vi "Get_Sampling_Info.vi"() -> (0 "Channel Values":string[](array[string]), 1 "Channel Names":string[](array[string]))   [LabVIEW 2011]
uses:
  Anemometry Sub Vis/Controls/Instrument_Array.ctl
  Anemometry Sub Vis/Globals/Meas_global.vi
  Anemometry Sub Vis/Globals/LDA_meas_global_1.vi
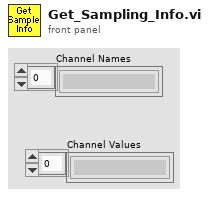
[diagram p1: front panel]
types:
  T1 = typedef "Instrument_Array.ctl" = enum16{"PWA", "LDA", "Analogue"}
  T2 = typedef "Analysis_info_cluster.ctl" = cluster{"Colour":u32, "Inst type":T3, "Inst name":string, "Symbol":string, "Code name":string, "Extra Info":string, "Inst Array":T1, "Extra Titles":string[], "Extra Values":string[], "Eng Values":dbl[], "Time (ms)":dbl[], "Voltage":dbl[], "U":dbl, "u^2":dbl, "u^3":dbl, "u^4":dbl, "Skew_u":dbl, "Kurt_u":dbl, "Sd Error in Mean":dbl, "% u'/U":dbl, "X":dbl, "Y":dbl, "Z":dbl, "Spectra":T4, "Autocorrelation":T4, "Timescale integral to 25%":dbl, "Sd Error in Variance":dbl, "Calib File":path, "Calib Constants":dbl[], "Histogram":T4, "Output Position":bool, "Full Stats":bool, "Weighting":dbl[], "Av Sampling Rate":dbl, "Av No of Samples":dbl, "Total Meas Time (s)":dbl}
  T3 = typedef "Inst_type.ctl" = enum16{"Propeller anemometer", "Raw voltage", "Pressure Transducer", "Pitot-static tube", "Preston tube", "Hot wire", "Cross wire 1", "Cross wire 2", "Generic Linear", "Generic Polynomial", "Generic BackPoly", "Fast FID", "Thermocouple", "Cold wire", "Pulsed Wire", "LDA Vel", "LDA Tran time", "LDA Arr time"}
  T4 = typedef "XY_Plot_Cluster.ctl" = cluster{"First Name":string, "Second Name":string, "X axis name":string, "Y axis name":string, "X array":dbl[], "Y array":dbl[]}
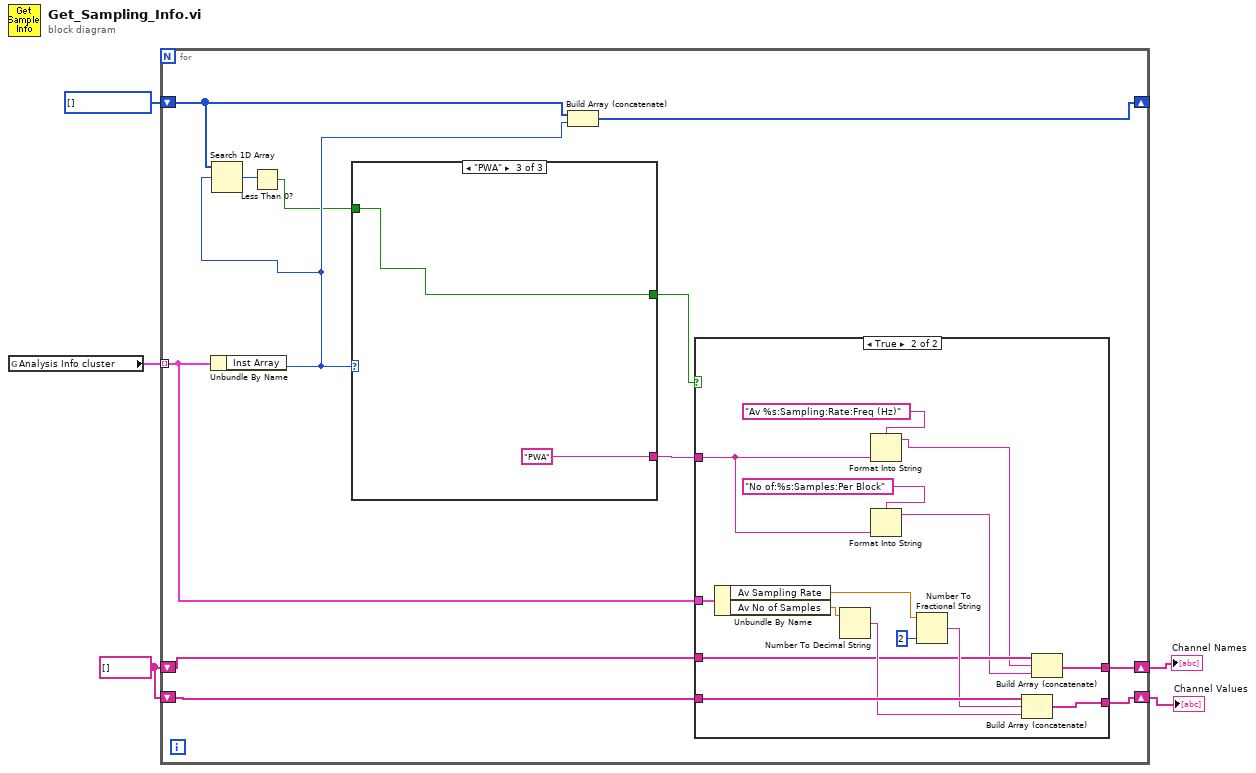
[diagram p0: block diagram]
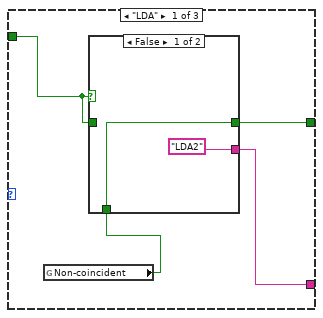
[diagram p3: hidden frame]
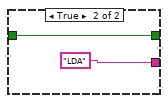
[diagram p4: hidden frame]
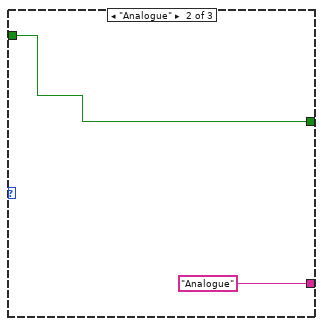
[diagram p5: hidden frame]
diagram:
  w3 = string[] []
  w4 = T1[] [] items=["PWA", "LDA", "Analogue"]
  n1 = global read "Meas_global.vi" "Analysis Info cluster"() -> (w5:T2[])
  n2 = for {
    shift-right: [w17] -> _
    shift-left: w4 -> [w16]
    tunnel: w5 -> [w11] mode=indexing
    shift-right: [w6] -> w1
    shift-left: w3 -> [w7]
    shift-right: [w8] -> w2
    shift-left: w3 -> [w9]
    n3 = Unbundle By Name(w11) -> ("Inst Array"=w15:T1)
    n4 = Search 1D Array(1D array=w16, element=w15) -> (index of element=w14:i32)  [unwired: 1 in]
    n5 = Less Than 0?(x=w14) -> (x < 0?=w13:bool)
    n6 = case shown="\"PWA\"" w15 {
      tunnel: w13 -> [w37 w44 w46]
      tunnel: [w38 w44 w46] -> w12
      tunnel: [w36 "Analogue" "PWA"] -> w10
      frame "LDA" {
        n7 = global read "LDA_meas_global_1.vi" "Non-coincident"() -> (w35:bool)
        n8 = case shown="False" w37 {
          tunnel: [w40 w42] -> w38
          tunnel: w37 -> [_ w42]
          tunnel: ["LDA2" "LDA"] -> w36
          tunnel: w35 -> [w40 _]
          frame False {
          }
          frame True {
          }
        }
      }
      frame "Analogue" {
      }
      frame "PWA" {
      }
    }
    n9 = Build Array (concatenate)(w16, w15) -> (w17:T1[])
    n10 = case shown="True" w12 {
      tunnel: w11 -> [_ w34]
      tunnel: w10 -> [_ w21]
      tunnel: w9 -> [w18 w31]
      tunnel: [w18 w30] -> w8
      tunnel: w7 -> [w19 w25]
      tunnel: [w19 w24] -> w6
      frame False {
      }
      frame True {
        n11 = Unbundle By Name(w34) -> ("Av Sampling Rate"=w28:dbl, "Av No of Samples"=w27:dbl)
        n12 = Number To Decimal String(number=w27) -> (decimal integer string=w26:string)  [unwired: 1 out]
        n13 = Format Into String(format string="Av %s:Sampling:Rate:Freq (Hz)", w21) -> (resulting string=w23:string)  [unwired: 2 in, 1 out]
        n14 = Format Into String(format string="No of:%s:Samples:Per Block", w21) -> (resulting string=w20:string)  [unwired: 2 in, 1 out]
        n15 = Number To Fractional String(number=w28, precision (6)=i16 2) -> (F-format string=w29:string)  [unwired: 2 out]
        n16 = Build Array (concatenate)(w31, w29, w26) -> (w30:string[])
        n17 = Build Array (concatenate)(w25, w23, w20) -> (w24:string[])
      }
    }
  }
  "Channel Names" <- w1
  "Channel Values" <- w2
